vi "声卡测试.vi"() -> ()   [LabVIEW 2018]
uses:
  <vilib>/Analysis/3filter.llb/Filter Passband Type.ctl
  <vilib>/measure/maresamp.llb/Resample Waveform (continuous).vi
  <vilib>/Analysis/3filter.llb/Butterworth Filter (DBL).vi
  <vilib>/express/express analysis/Spectral/Block/exnSpectralBlock spectral measurements peak poly.vi
  <vilib>/express/express analysis/Spectral/Block/exnSpectralBlock spectral measurements peak WFM.vi
  <vilib>/express/express analysis/Spectral/XNode/ExpressSpectralMeasurementsBlockNode.xnode
  <vilib>/measure/NI_MABase.lvlib
  <vilib>/Analysis/NI_AALPro.lvlib
  <vilib>/measure/NI_MAPro.lvlib
  <vilib>/Analysis/NI_AALBase.lvlib
panel:
  in  "选项卡控件":enum32{"时域", "频域"}(tab)
  out "调制信号":waveform(dbl)(graph)
  out "解调":waveform(dbl)[](graph)
  out "解调（细节）":waveform(dbl)[](graph)
  out "已调频域":cluster{"f0":dbl, "df":dbl, "magnitude":dbl[]}(graph)
  out "滤波后频域":cluster{"f0":dbl, "df":dbl, "magnitude":dbl[]}(graph)
  in  "低通滤波fl":dbl=80000.0
  in  "kf(Hz/V)":dbl=50000.0
  out "实验系统采样参数\n采样频率fs，采样数Ns":cluster{dbl, dbl} {"?" format="%#_6f"; "?" format="%#_6f"}
  in  "载波信号":cluster{"fc(Hz)":dbl, "Ac(V)":dbl}={"fc(Hz)"=50000.0, "Ac(V)"=0.3}
  in  "An(V)":dbl=0.02
  in  "Sample rate (Hz)":dbl=5000.0 caption="声卡采样率(Hz)"
  in  "Duration (s)":dbl=2.0 caption="持续时间(s)"
  # "人声频率在100-500Hz"
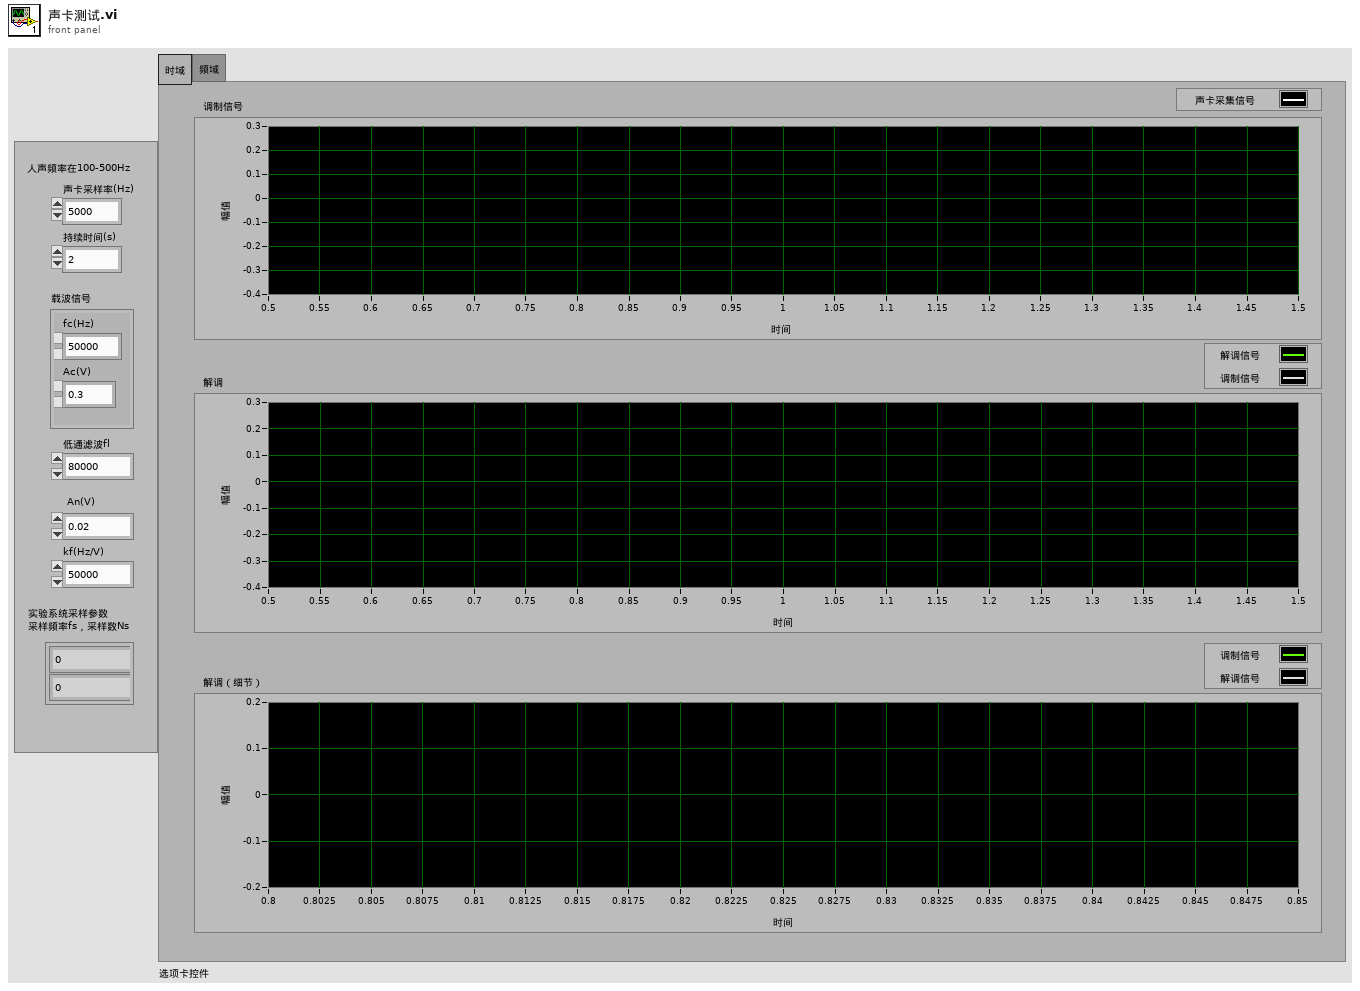
[diagram p1: front panel]
types:
  T1 = typedef "NI_AALBase.lvlib/Filter Passband Type.ctl" = enum32{"Lowpass", "Highpass", "Bandpass", "Bandstop"}
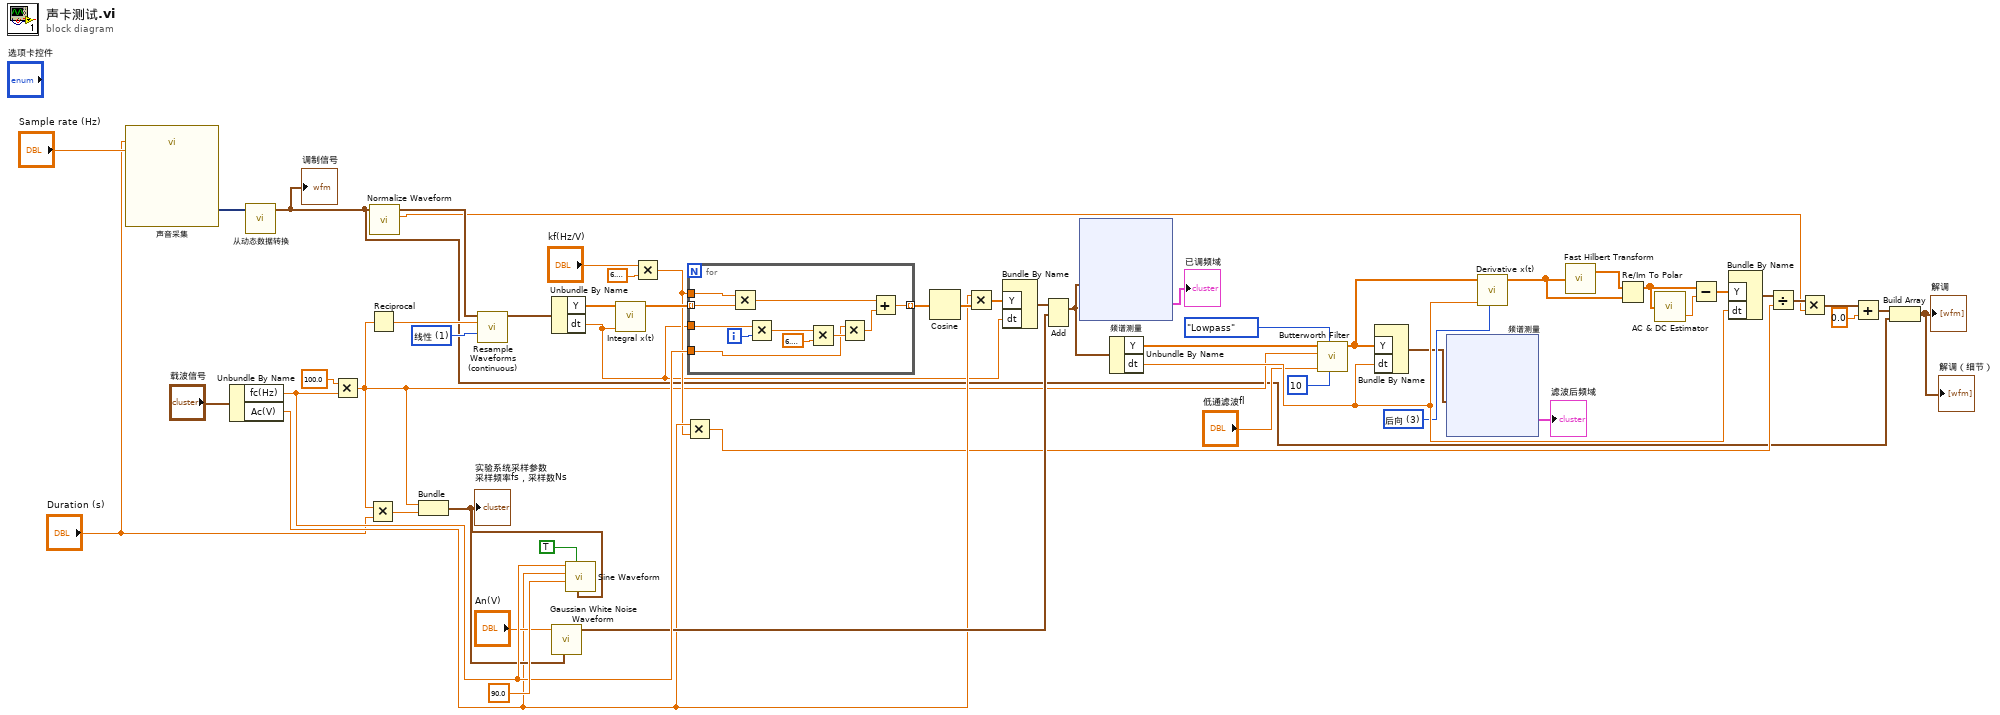
[diagram p0: block diagram]
diagram:
  w21 = u16 1 items=["强制", "线性", "样条", "FIR滤波"] ("interpolation mode")
  w32 = u16 3 items=["二阶中心", "四阶中心", "前向", "后向"] ("method")
  n1 = call "声音采集"("Duration (s)"="Duration (s)", "Sample rate (Hz)"="Sample rate (Hz)") -> ("Data"=w16:dynamicdata)  [unwired: 16 in, 1 out]
  n2 = Unbundle By Name("载波信号") -> ("fc(Hz)"=w47:dbl, "Ac(V)"=w28:dbl)
  n3 = call "从动态数据转换"("Dynamic Data Type"=w16) -> ("Waveform"=w3:waveform(dbl))  [unwired: 3 in]
  "调制信号" <- w3
  n4 = Multiply(x=100.0, y=w47) -> (x*y=w18:dbl)
  n5 = Multiply(x=w18, y="Duration (s)") -> (x*y=w19:dbl)
  n6 = Reciprocal(x=w18) -> (1/x=w17:dbl)
  n7 = call <vilib>:"Normalize Waveform.vi"("waveform in"=w3) -> ("scale"=w6:dbl, "normalized waveform"=w8:waveform(dbl))  [unwired: 7 in, 2 out]
  n8 = Bundle(w18, w19) -> (w42:cluster{dbl, dbl})  [unwired: 1 in]
  "实验系统采样参数\n采样频率fs，采样数Ns" <- w42
  n9 = call-poly <vilib>:"Resample Waveforms (continuous).vi"("waveform in"=w8, "dt"=w17, "interpolation mode"=w21) -> ("resampled waveform out"=w10:waveform(dbl))  [unwired: 8 in, 4 out]
  n10 = Unbundle By Name(w10) -> ("Y"=w15:dbl[], "dt"=w14:dbl)
  n11 = call <vilib>:"Gaussian White Noise Waveform.vi"("sampling info"=w42, "standard deviation"="An(V)") -> ("signal out"=w40:waveform(dbl))  [unwired: 8 in, 1 out]
  n12 = call <vilib>:"Sine Waveform.vi"("sampling info"=w42, "reset signal"=TRUE, "phase"=90.0, "amplitude"=w28, "frequency"=w47) -> ()  [unwired: 5 in, 2 out]
  n13 = call <vilib>:"Integral x(t).vi"("dt"=w14, "X"=w15) -> ("Integral X"=w48:dbl[])  [unwired: 8 in, 1 out]
  n14 = Multiply(x="kf(Hz/V)", y=6.283185307179586) -> (x*y=w22:dbl)
  n15 = Multiply(x=w28, y=w22) -> (x*y=w26:dbl)
  n16 = for {
    tunnel: w48 -> [w64] mode=indexing
    tunnel: w47 -> [w59]
    tunnel: [w56] -> w46 mode=indexing
    tunnel: w22 -> [w55]
    tunnel: w14 -> [w54]
    i -> [w63]
    n17 = Multiply(x=w55, y=w64) -> (x*y=w57:dbl)
    n18 = Multiply(x=w54, y=w63) -> (x*y=w61:dbl)
    n19 = Multiply(x=w61, y=6.283185307179586) -> (x*y=w60:dbl)
    n20 = Multiply(x=w59, y=w60) -> (x*y=w58:dbl)
    n21 = Add(x=w57, y=w58) -> (x+y=w56:dbl)
  }
  n22 = Cosine(x=w46) -> (cos(x)=w45:dbl[])
  n23 = Multiply(x=w28, y=w45) -> (x*y=w44:dbl[])
  n24 = Bundle By Name("Y"=w44, "dt"=w14) -> (w41:waveform(dbl))  [unwired: 1 in]
  n25 = Add(1:w40, 2:w41) -> (0:w37:waveform(dbl))  [unwired: 1 in, 1 out]
  n26 = xnode "频谱测量"("信号"=w37) -> ("FFT - （峰值）"=→"已调频域":cluster{"f0":dbl, "df":dbl, "magnitude":dbl[]})  [unwired: 1 in, 2 out]
  n27 = Unbundle By Name(w37) -> ("Y"=w36:dbl[], "dt"=w33:dbl)
  n28 = call-poly <vilib>:"Butterworth Filter.vi"("order"=10, "filter type"=Filter_Passband_Type."Lowpass", "low cutoff freq: fl"="低通滤波fl", "sampling freq: fs"=w18, "X"=w36) -> ("Filtered X"=w35:dbl[])  [unwired: 3 in, 1 out]
  n29 = Bundle By Name("Y"=w35, "dt"=w33) -> (w11:waveform(dbl))  [unwired: 1 in]
  n30 = xnode "频谱测量"("信号"=w11) -> ("FFT - （峰值）"=→"滤波后频域":cluster{"f0":dbl, "df":dbl, "magnitude":dbl[]})  [unwired: 1 in, 2 out]
  n31 = call <vilib>:"Derivative x(t).vi"("method"=w32, "dt"=w33, "X"=w35) -> ("dX/dt"=w25:dbl[])  [unwired: 7 in, 1 out]
  n32 = call <vilib>:"Fast Hilbert Transform.vi"("X"=w25) -> ("Hilbert{X}"=w34:dbl[])  [unwired: 1 out]
  n33 = Re/Im To Polar(2:w25, 3:w34) -> (1:w31:dbl[])  [unwired: 1 out]
  n34 = call <vilib>:"AC & DC Estimator.vi"("Signal (V)"=w31) -> ("DC estimate (V)"=w30:dbl)  [unwired: 1 out]
  n35 = Subtract(x=w31, y=w30) -> (x-y=w29:dbl[])
  n36 = Bundle By Name("Y"=w29, "dt"=w33) -> (w27:waveform(dbl))  [unwired: 1 in]
  n37 = Divide(x=w27, y=w26) -> (x/y=w7:waveform(dbl))
  n38 = Multiply(x=w7, y=w6) -> (x*y=w5:waveform(dbl))
  n39 = Add(x=w5, y=0.0) -> (x+y=w1:waveform(dbl))
  n40 = Build Array(w1, w3) -> (→"解调" →"解调（细节）":waveform(dbl)[])
